vi "Plot Format 1D Table.vi"(8 "Data 1D Table":cluster{"X":sgl[], "Y":sgl[]}, 11 "Table Ref":refnum<vi>) -> ()   [LabVIEW 2016]
uses:
  <vilib>/Utility/miscctls.llb/LVRowAndColumnTypeDef.ctl
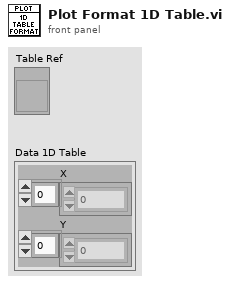
[diagram p1: front panel]
types:
  T1 = typedef "LVRowAndColumnTypeDef.ctl" = cluster{"Row":i32, "Column":i32}
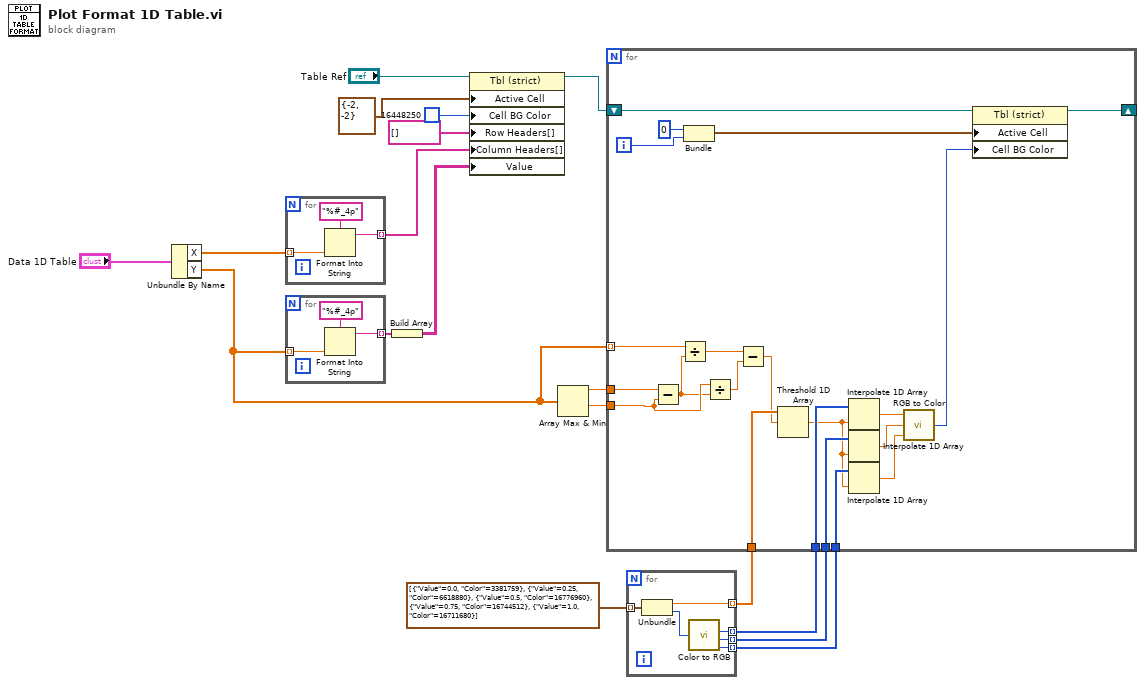
[diagram p0: block diagram]
diagram:
  n1 = Unbundle By Name("Data 1D Table") -> ("X"=w18:sgl[], "Y"=w6:sgl[])
  n2 = for {
    tunnel: w18 -> [w21] mode=indexing
    tunnel: [w19] -> w7 mode=indexing
    n3 = Format Into String(format string="%#_4p", w21) -> (resulting string=w19:string)  [unwired: 2 in, 1 out]
  }
  n4 = for {
    tunnel: w6 -> [w24] mode=indexing
    tunnel: [w22] -> w17 mode=indexing
    n5 = Format Into String(format string="%#_4p", w24) -> (resulting string=w22:string)  [unwired: 2 in, 1 out]
  }
  n6 = Build Array(w17) -> (w5:string[][])
  n7 = property on="Property Node" class="Tbl (strict)"(reference="Table Ref", "Active Cell"=T1 {"Row"=-2, "Column"=-2} ("Active Cell:Active Cell"), "Cell BG Color"=u32 16448250 ("Active Cell:Cell Background Color"), "Row Headers[]"=string[] [] ("Row Header Strings[]"), "Column Headers[]"=w7, "Value"=w5) -> (reference out=w14:refnum<vi>)  [unwired: 1 in, 1 out]
  n8 = Array Max & Min(array=w6) -> (max value=w16:sgl, min value=w15:sgl)  [unwired: 2 out]
  n9 = for {
    tunnel: cluster{"Value":sgl, "Color":u32}[] [{"Value"=0.0, "Color"=3381759}, {"Value"=0.25, "Color"=6618880}, {"Value"=0.5, "Color"=16776960}, {"Value"=0.75, "Color"=16744512}, {"Value"=1.0, "Color"=16711680}] -> [w30] mode=indexing
    tunnel: [w28] -> w13 mode=indexing
    tunnel: [w27] -> w12 mode=indexing
    tunnel: [w26] -> w11 mode=indexing
    tunnel: [w25] -> w10 mode=indexing
    n10 = Unbundle(w30) -> ("Value"=w25:sgl, "Color"=w29:u32)
    n11 = call <vilib>:"Color to RGB.vi"("Color"=w29) -> ("R"=w28:u8, "G"=w27:u8, "B"=w26:u8)  [unwired: 1 out]
  }
  n12 = for {
    tunnel: w16 -> [w51]
    tunnel: w15 -> [w50]
    tunnel: w6 -> [w49] mode=indexing
    shift-right: [w47] -> _
    shift-left: w14 -> [w48]
    tunnel: w13 -> [w46]
    tunnel: w12 -> [w45]
    tunnel: w11 -> [w44]
    tunnel: w10 -> [w43]
    i -> [w33]
    n13 = Subtract(x=w51, y=w50) -> (x-y=w42:sgl)
    n14 = Divide(x=w49, y=w42) -> (x/y=w41:sgl)
    n15 = Bundle(0, w33) -> (w36:cluster{i32, i32})  [unwired: 1 in]
    n16 = Divide(x=w50, y=w42) -> (x/y=w40:sgl)
    n17 = Subtract(x=w41, y=w40) -> (x-y=w31:sgl)
    n18 = Threshold 1D Array(2:w31, 3:w43) -> (0:w32:sgl)  [unwired: 1 in]
    n19 = Interpolate 1D Array(1:w32, 2:w46) -> (0:w37:dbl)
    n20 = Interpolate 1D Array(1:w32, 2:w45) -> (0:w38:dbl)
    n21 = Interpolate 1D Array(1:w32, 2:w44) -> (0:w39:dbl)
    n22 = call <vilib>:"RGB to Color.vi"("B"=w39, "G"=w38, "R"=w37) -> ("Color"=w35:u32)
    n23 = property on="Property Node" class="Tbl (strict)"(reference=w48, "Active Cell"=w36, "Cell BG Color"=w35) -> (reference out=w47:refnum<vi>)  [unwired: 1 in, 1 out]
  }
